vi "Read Group ID.vi"(8 "Error In":errorcluster, 11 "SFTP Attributes In":refnum<class "SFTP Attributes.lvclass">) -> (0 "Error Out":errorcluster, 2 "ID":u32, 3 "SFTP Attribute Out":refnum<class "SFTP Attributes.lvclass">)   [LabVIEW 2018, in "Toolkit.lvlib" / "SFTP Attributes.lvclass"]
uses:
  SFTP Attributes.lvclass
  SFTP Attributes.lvclass/SFTP Attributes.ctl
  SSH/SSH.lvclass/SSH.ctl
  Toolkit.lvlib
  SSH/SSH.lvclass
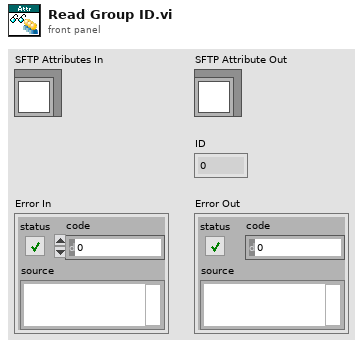
[diagram p1: front panel]
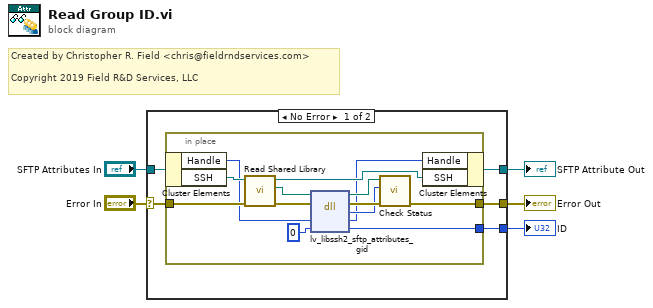
[diagram p0: block diagram]
diagram:
  # "Created by Christopher R. Field <chris@fieldrndservices.com>\n\nCopyright 2019 Field R&D Services, LLC"
  n1 = case shown="No Error" "Error In" {
    selector: "Error In" -> [w9 w25]
    tunnel: [w7 w25] -> w4
    tunnel: "SFTP Attributes In" -> [w10 w24]
    tunnel: [w8 w24] -> w2
    tunnel: [w6 _] -> w1
    frame No Error {
      n2 = in-place {
        in-place-border: w9 -> [w16]
        in-place-border: [w13] -> w7
        in-place-border: [w11] -> w6
        n3 = in-place-cluster #1(w10) -> ("Handle"=w15:u64, "SSH"=w20:refnum<class "SSH.lvclass">)
        n4 = call "Read Shared Library.vi"("Error In"=w16, "SSH In"=w20) -> ("Error Out"=w17:errorcluster, "lv-libssh2 Shared Library"=w18:path, "SSH Out"=w19:refnum<class "SSH.lvclass">)  [unwired: 7 in]
        n5 = dll-call lib="lv-libssh2.*" fn="lv_libssh2_sftp_attributes_gid"(path in=w18, error in=w17, "handle"=w15, "gid"=u32 0 ("flags")) -> (path out=w22:path, error out=w23:errorcluster, "status"=w21:i32, "handle"=w14:u64, "gid"=w11:u32)  [unwired: 1 in]
        n6 = call "Check Status.vi"("Error In"=w23, "Status"=w21, "lv-libssh2 Shared Library In"=w22) -> ("Error Out"=w13:errorcluster)  [unwired: 7 in, 1 out]
        n7 = in-place-cluster #1("Handle"=w14, "SSH"=w19) -> (w8:refnum<class "SFTP Attributes.lvclass">)
      }
    }
    frame Error {
    }
  }
  "Error Out" <- w4
  "SFTP Attribute Out" <- w2
  "ID" <- w1
